vi "get_addressee.vi"(8 "error in (no error)":errorcluster, 11 "HGF_Visitor":refnum<class "HGF_Visitor.lvclass">) -> (0 "error out":errorcluster, 2 "addressee":string, 3 "dup HGF_Visitor":refnum<class "HGF_Visitor.lvclass">)   [LabVIEW 2014, in "HGF_BaseClasses.lvlib" / "HGF_Visitor.lvclass"]
doc: "Returns name of object that should recieve this visitor."
uses:
  HGF_Visitor.lvclass
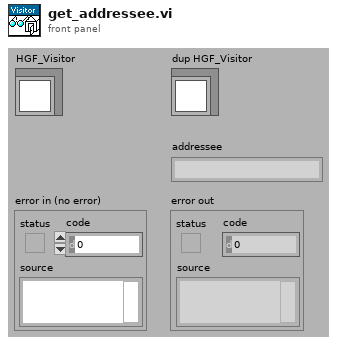
[diagram p1: front panel]
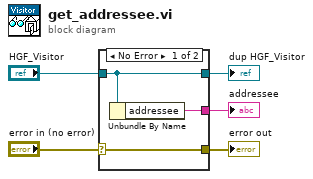
[diagram p0: block diagram]
diagram:
  n1 = case shown="No Error" "error in (no error)" {
    selector: "error in (no error)" -> [w8 w9]
    tunnel: [w8 w9] -> w4
    tunnel: [w7 w10] -> w2
    tunnel: "HGF_Visitor" -> [w7 w10]
    tunnel: [w6 _] -> w1
    frame No Error {
      n2 = Unbundle By Name(w7) -> ("addressee"=w6:string)
    }
    frame Error {
    }
  }
  "error out" <- w4
  "dup HGF_Visitor" <- w2
  "addressee" <- w1
